vi "AssignSample.vi"(6 "PMT state":bool=TRUE, 8 "Current laser state":bool=TRUE, 9 "Previous laser state":bool=TRUE, 10 "Photon counters in":T2=[0, 0], 11 "Region selector in":T1 max=1) -> (2 "Photon counters out":T2, 3 "Region selector out":T1 max=1)   [LabVIEW 2012]
uses:
  RegionalPhotonCounters.ctl
  RegionSelector.ctl
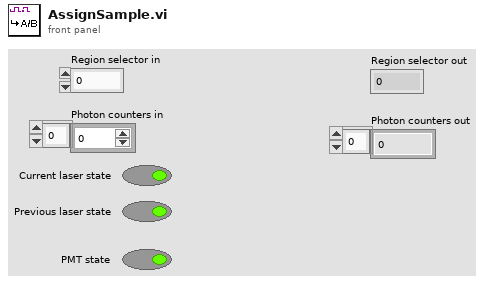
[diagram p1: front panel]
types:
  T1 = typedef "RegionSelector.ctl" = i16
  T2 = typedef "RegionalPhotonCounters.ctl" = u16[]
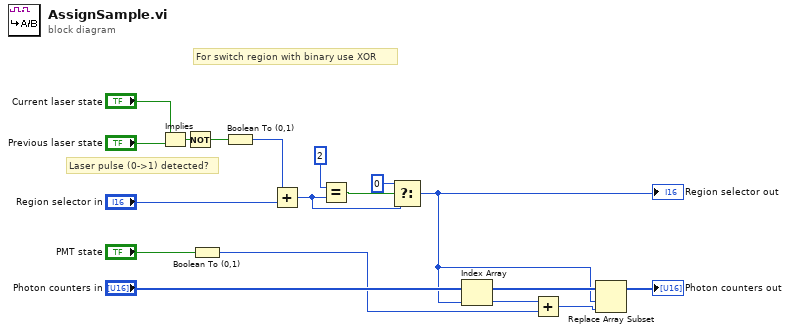
[diagram p0: block diagram]
diagram:
  # "For switch region with binary use XOR"
  # "Laser pulse (0->1) detected?"
  n1 = Implies(1:"Previous laser state", 2:"Current laser state") -> (0:w15:bool)
  n2 = Not(x=w15) -> (.not. x?=w13:bool)
  n3 = Boolean To (0,1)(Boolean="PMT state") -> (0, 1=w4:i16)
  n4 = Boolean To (0,1)(Boolean=w13) -> (0, 1=w3:i16)
  n5 = Add(x=w3, y="Region selector in") -> (x+y=w9:T1)
  n6 = Equal?(x=T1 2, y=w9) -> (x = y?=w10:bool)
  n7 = Select(t=T1 0, s=w10, f=w9) -> (s? t:f=w6:T1)
  "Region selector out" <- w6
  n8 = Index Array(array="Photon counters in", index=w6) -> (element=w5:u16)
  n9 = Add(x=w5, y=w4) -> (x+y=w2:u16)
  n10 = Replace Array Subset(array="Photon counters in", new element=w2, index=w6) -> (→"Photon counters out":T2)
